vi "SampleGetPositionAllSlavesyes.vi"() -> ()   [LabVIEW 2021]
panel:
  out "Output:":string
  out "DeviceKey List Out":string[](array[string])
  out "error out":errorcluster
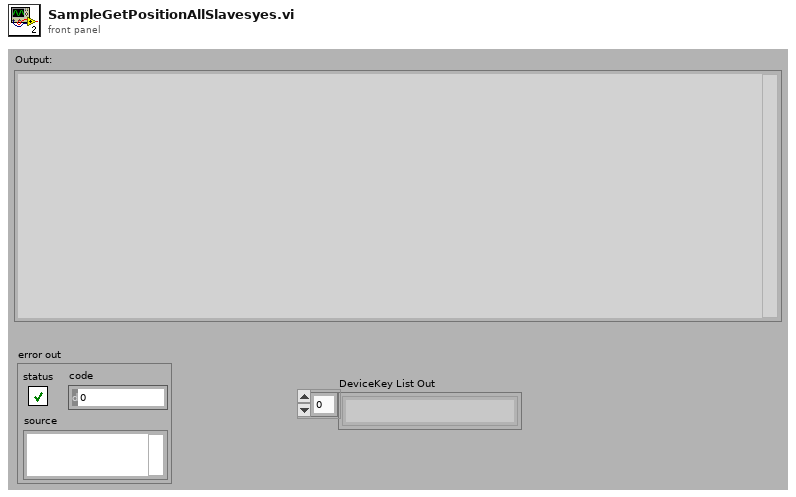
[diagram p1: front panel]
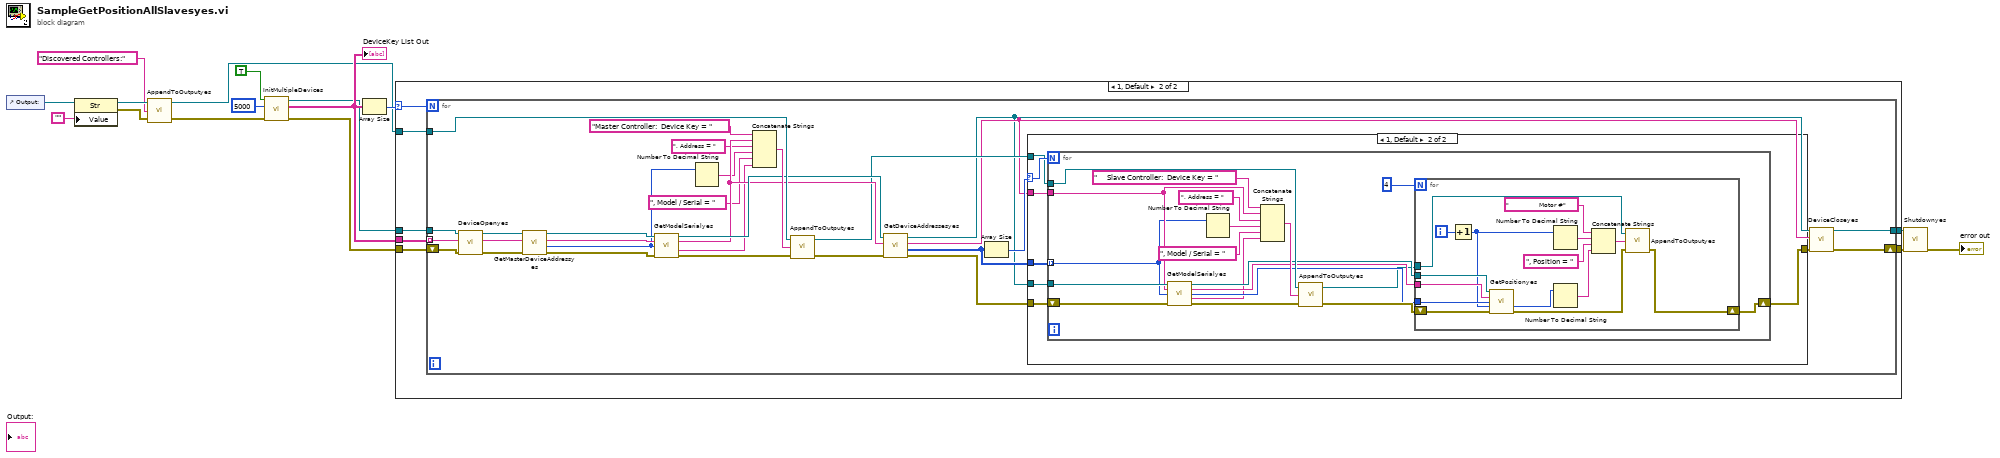
[diagram p0: block diagram]
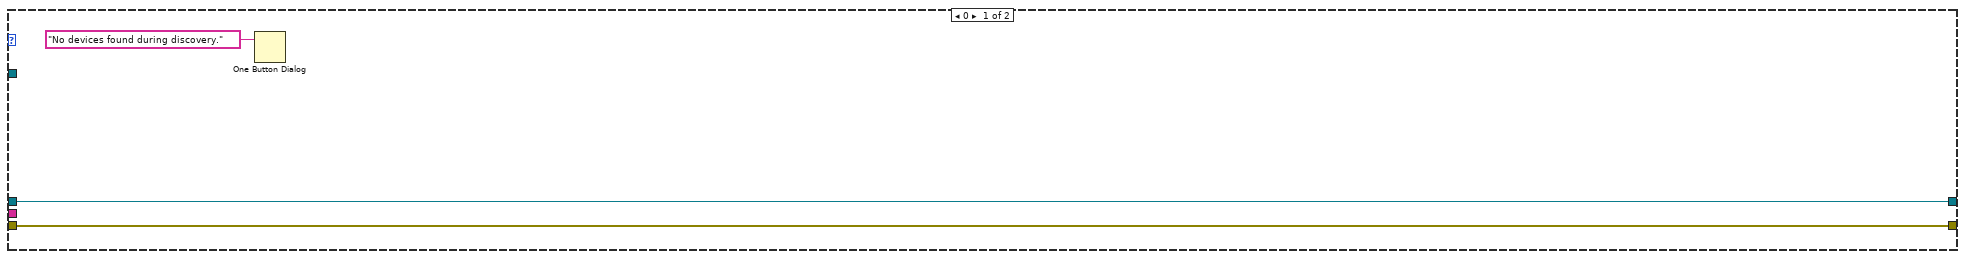
[diagram p2: hidden frame]
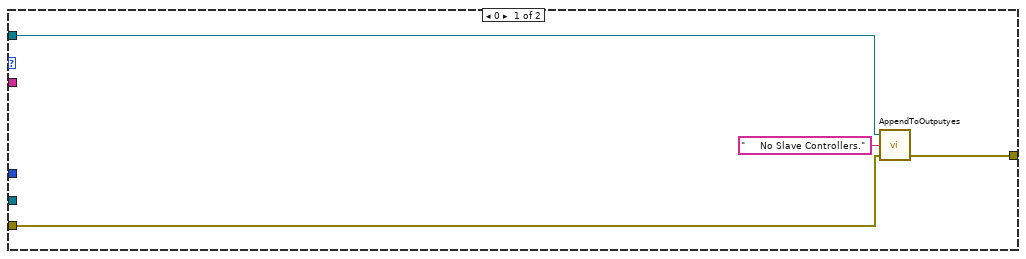
[diagram p3: hidden frame]
diagram:
  n1 = control-ref of="Output:"() -> (w7:refnum<vi>)
  n2 = property class="Str"(reference=w7, "Value"="") -> (reference out=w5:refnum<vi>, error out=w4:errorcluster)  [unwired: 1 in]
  n3 = call "AppendToOutputyes.vi"("error in"=w4, "Input String"="Discovered Controllers:", "Output Refnum In"=w5) -> ("error out"=w3:errorcluster, "Output Refnum Out"=w1:refnum<vi>)  [unwired: 1 in]
  n4 = call "InitMultipleDevices.vi"("error in (no error)"=w3, "msecDelayForDiscovery"=5000, "logging"=TRUE) -> ("error out"=w10:errorcluster, "DeviceKey List Out"=w12:string[], "CmdLib Out"=w11:refnum<k24>)  [unwired: 2 in]
  "DeviceKey List Out" <- w12
  n5 = Array Size(array=w12) -> (size(s)=w13:i32)
  n6 = case shown="1, Default" w13 {
    selector: w13 -> [_ w26]
    tunnel: w12 -> [_ w25]
    tunnel: w11 -> [w18 w24]
    tunnel: w10 -> [w19 w23]
    tunnel: [w19 w22] -> w9
    tunnel: [w18 w21] -> w8
    tunnel: w1 -> [_ w20]
    frame 0 {
      n7 = One Button Dialog(message="No devices found during discovery.") -> ()  [unwired: 1 in, 1 out]
    }
    frame 1, Default {
      n8 = for {
        N: w26 -> [_]
        tunnel: w25 -> [w54] mode=indexing
        tunnel: w24 -> [w56]
        tunnel: [w55] -> w21
        tunnel: w20 -> [w51]
        shift-right: [w52] -> w22
        shift-left: w23 -> [w53]
        n9 = call "DeviceOpenyes.vi"("error in (no error)"=w53, "DeviceKey In"=w54, "CmdLib In"=w56) -> ("error out"=w45:errorcluster, "DeviceKey Out"=w46:string, "CmdLib Out"=w47:refnum<k24>)  [unwired: 2 in]
        n10 = call "GetMasterDeviceAddressyes.vi"("error in (no error)"=w45, "DeviceKey In"=w46, "CmdLib In"=w47) -> ("error out"=w42:errorcluster, "Device Address"=w27:i32, "DeviceKey Out"=w41:string, "CmdLib Out"=w40:refnum<k24>)  [unwired: 1 in]
        n11 = call "GetModelSerialyes.vi"("CmdLib In"=w40, "DeviceKey In"=w41, "Device Address In"=w27, "error in (no error)"=w42) -> ("CmdLib Out"=w43:refnum<k24>, "DeviceKey Out"=w39:string, "Model / Serial"=w35:string, "error out"=w44:errorcluster)  [unwired: 7 in, 1 out]
        n12 = Number To Decimal String(number=w27) -> (decimal integer string=w37:string)  [unwired: 1 in]
        n13 = Concatenate Strings("Master Controller:  Device Key = " ("string"), w39, ", Address = " ("string"), w37, ", Model / Serial = " ("string"), w35) -> (w50:string)
        n14 = call "AppendToOutputyes.vi"("error in"=w44, "Input String"=w50, "Output Refnum In"=w51) -> ("error out"=w48:errorcluster, "Output Refnum Out"=w33:refnum<vi>)  [unwired: 1 in]
        n15 = call "GetDeviceAddressesyes.vi"("error in (no error)"=w48, "DeviceKey In"=w39, "CmdLib In"=w43) -> ("error out"=w32:errorcluster, "Device Addresses"=w30:i32[], "DeviceKey Out"=w29:string, "CmdLib Out"=w28:refnum<k24>)  [unwired: 1 in]
        n16 = Array Size(array=w30) -> (size(s)=w34:i32)
        n17 = case shown="1, Default" w34 {
          selector: w34 -> [_ w67]
          tunnel: w33 -> [w59 w63]
          tunnel: w32 -> [w58 w61]
          tunnel: [w57 w64] -> w31
          tunnel: w30 -> [_ w66]
          tunnel: w29 -> [_ w65]
          tunnel: w28 -> [_ w62]
          frame 0 {
            n18 = call "AppendToOutputyes.vi"("error in"=w58, "Input String"="     No Slave Controllers.", "Output Refnum In"=w59) -> ("error out"=w57:errorcluster)  [unwired: 1 in, 1 out]
          }
          frame 1, Default {
            n19 = for {
              N: w67 -> [_]
              tunnel: w66 -> [w78] mode=indexing
              tunnel: w65 -> [w79]
              tunnel: w63 -> [w82]
              tunnel: w62 -> [w80]
              shift-right: [w73] -> w64
              shift-left: w61 -> [w77]
              n20 = call "GetModelSerialyes.vi"("CmdLib In"=w80, "DeviceKey In"=w79, "Device Address In"=w78, "error in (no error)"=w77) -> ("CmdLib Out"=w75:refnum<k24>, "DeviceKey Out"=w76:string, "Device Address Out"=w72:i32, "Model / Serial"=w70:string, "error out"=w69:errorcluster)  [unwired: 7 in]
              n21 = Number To Decimal String(number=w78) -> (decimal integer string=w84:string)  [unwired: 1 in]
              n22 = Concatenate Strings("     Slave Controller:  Device Key = " ("string"), w79, ", Address = " ("string"), w84, ", Model / Serial = " ("string"), w70) -> (w81:string)
              n23 = call "AppendToOutputyes.vi"("error in"=w69, "Input String"=w81, "Output Refnum In"=w82) -> ("error out"=w74:errorcluster, "Output Refnum Out"=w71:refnum<vi>)  [unwired: 1 in]
              n24 = for {
                N: 4 ("f") -> [_]
                tunnel: w76 -> [w101]
                tunnel: w75 -> [w100]
                tunnel: w72 -> [w98]
                tunnel: w71 -> [w96]
                shift-right: [w97] -> w73
                shift-left: w74 -> [w99]
                i -> [w92]
                n25 = Increment(x=w92) -> (x+1=w88:i32)
                n26 = call "GetPositionyes.vi"("CmdLib In"=w100, "DeviceKey In"=w101, "Device Address In"=w98, "Motor"=w88, "error in (no error)"=w99) -> ("Position"=w91:i32, "error out"=w87:errorcluster)  [unwired: 6 in, 3 out]
                n27 = Number To Decimal String(number=w88) -> (decimal integer string=w93:string)  [unwired: 1 in]
                n28 = Number To Decimal String(number=w91) -> (decimal integer string=w90:string)  [unwired: 1 in]
                n29 = Concatenate Strings("               Motor #" ("Input String"), w93, ", Position = " ("string"), w90) -> (w94:string)
                n30 = call "AppendToOutputyes.vi"("error in"=w87, "Input String"=w94, "Output Refnum In"=w96) -> ("error out"=w97:errorcluster)  [unwired: 1 in, 1 out]
              }
            }
          }
        }
        n31 = call "DeviceCloseyes.vi"("error in (no error)"=w31, "DeviceKey In"=w29, "CmdLib In"=w28) -> ("error out"=w52:errorcluster, "CmdLib Out"=w55:refnum<k24>)  [unwired: 2 in, 1 out]
      }
    }
  }
  n32 = call "Shutdownyes.vi"("error in (no error)"=w9, "CmdLib In"=w8) -> ("error out"=→"error out":errorcluster)  [unwired: 4 in, 1 out]
